vi "GymkhanaRetryRoll.vi"(9 "inputRetry":bool, 10 "inputLabTIme(ms)":i64, 11 "inputGymkhanaSubLooptate":T1) -> (2 "outputLabTime(ms)":i64, 3 "outputGymkhanaSubLooptate":T1)   [LabVIEW 2020]
uses:
  Control/GymkhanaSubLoopState.ctl
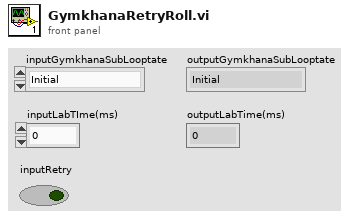
[diagram p1: front panel]
types:
  T1 = typedef "GymkhanaSubLoopState.ctl" = enum16{"Initial", "Ready", "Running", "FinishRunning", "DNF"}
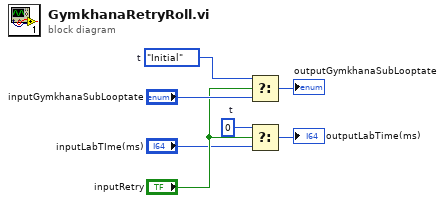
[diagram p0: block diagram]
diagram:
  w2 = i64 0  # t
  w5 = GymkhanaSubLoopState."Initial"  # t
  n1 = Select(t=w5, s="inputRetry", f="inputGymkhanaSubLooptate") -> (s? t:f=→"outputGymkhanaSubLooptate":T1)
  n2 = Select(t=w2, s="inputRetry", f="inputLabTIme(ms)") -> (s? t:f=→"outputLabTime(ms)":i64)
